vi "Call Subpanel VI.vi"(8 "error in (no error)":errorcluster, 10 "VI Refnum":refnum<vi>, 11 "GaugeController Configuration in":refnum<class "GaugeController Configuration.lvclass">) -> (0 "error out":errorcluster, 3 "GaugeController Configuration out":refnum<class "GaugeController Configuration.lvclass">)   [LabVIEW 2016, in "Hardware.lvlib" / "GaugeController.lvlib" / "GaugeController Configuration.lvclass"]
uses:
  <userlib>/Common Components/Hardware/GaugeController/GaugeController Config/GaugeController Configuration.lvclass
  <userlib>/Configuration Dialog Actor/Configuration.lvclass
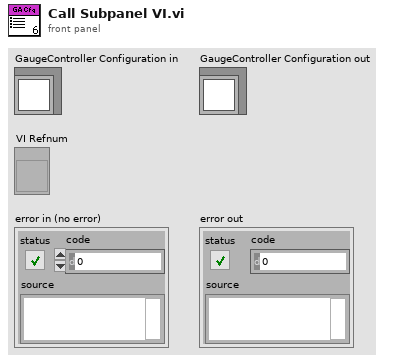
[diagram p1: front panel]
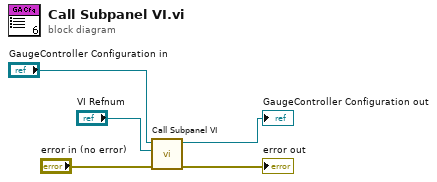
[diagram p0: block diagram]
diagram:
  n1 = call-parent "Call Subpanel VI.vi"("error in (no error)"="error in (no error)", "VI Refnum"="VI Refnum", "Configuration in"="GaugeController Configuration in") -> ("error out"=→"error out":errorcluster, "Configuration out"=→"GaugeController Configuration out":refnum<class "GaugeController Configuration.lvclass">)  [unwired: 7 in]
